vi "Renishaw-XL80_GetIsConnect.vi"(8 "error in (no error)":errorcluster, 11 "Renishaw-XL80_EMU in":refnum<class "Renishaw-XL80_EMU.lvclass">) -> (0 "error out":errorcluster, 2 "IsConnected":bool, 3 "Renishaw-XL80_EMU out":refnum<class "Renishaw-XL80_EMU.lvclass">)   [LabVIEW 2024, in "Renishaw-XL80_EMU.lvclass"]
doc: "This read only property returns VARIANT_TRUE if the client has connected to a DX10 and returns VARIANT_FALSE otherwise.\n\nDefinition\nHRESULT\nget_IsConnected(\n [out, retval] VARIANT_BOOL* pVal\n);\n\nParameters\npVal\nA variable that will be set to VARIANT_TRUE or VARIANT_FALSE. \nComments\nIf this property sets pVal to VARIANT_FALSE then this indicates that either the client has not called Connect, or that the client called Connect and the method failed to find an available DX10. The property will also set pVal to VARIANT_FALSE if the client has previously called Disconnect.\n\nThe property will normally return an HRESULT of S_OK. However, it will return E_POINTER if the client supplies a null pointer for pVal."
uses:
  Renishaw-XL80_EMU.lvclass
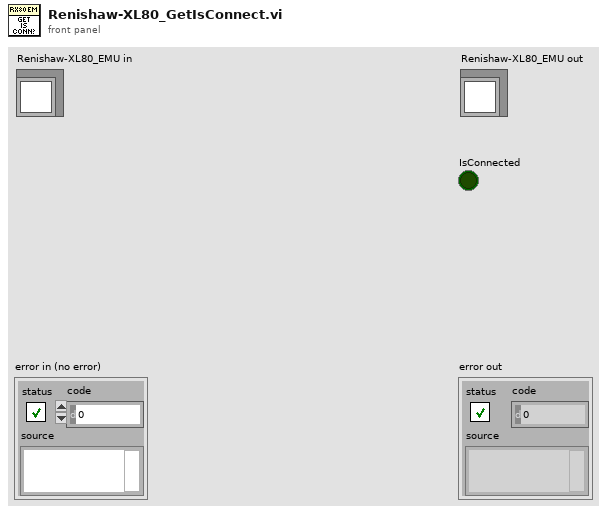
[diagram p1: front panel]
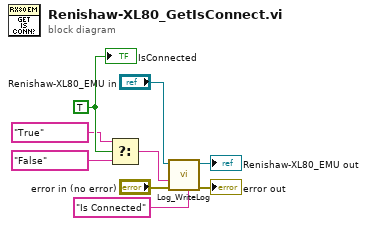
[diagram p0: block diagram]
diagram:
  w4 = TRUE ("IsConnected")
  n1 = Select(t="True" ("Additional text"), s=w4, f="False" ("Additional text")) -> (s? t:f=w1:string)
  n2 = call-dynamic "Log_WriteLog.vi"("Additional text"="Is Connected", "error in (no error)"="error in (no error)", "Response"=w1, "Log in"="Renishaw-XL80_EMU in") -> ("error out"=→"error out":errorcluster, "Log out"=→"Renishaw-XL80_EMU out":refnum<class "Renishaw-XL80_EMU.lvclass">)  [unwired: 6 in]
  "IsConnected" <- w4
